vi "set gain and exp time for Basler acA2500-60um (SubVI).vi"(7 "Acquisition Control::Exposure Time":dbl, 8 "error in (no error)":errorcluster, 9 "Analog Control::Gain":dbl, 10 "Session Out":T2, 11 "Refnum in":T1) -> (0 "error out":errorcluster, 3 "Refnum out":T1)   [LabVIEW 2024]
uses:
  <vilib>/userDefined/High Color/IMAQdx.ctl
  <vilib>/vision/Image Controls.llb/IMAQ Image.ctl
  <resource>/objmgr/imaqdx.rc
  <vilib>/vision/driver/NI_Vision_Acquisition_Software.lvlib
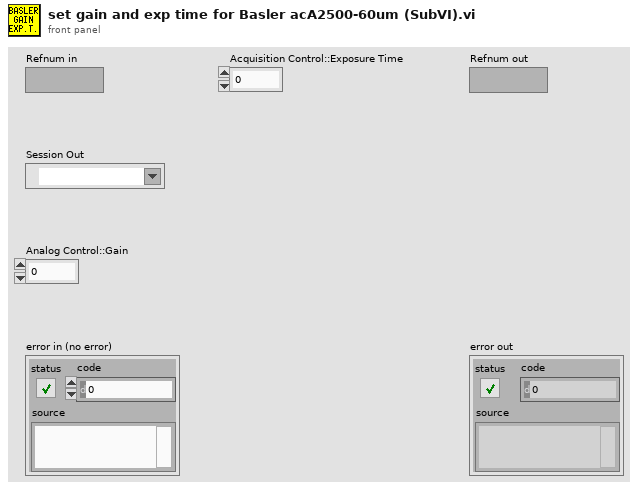
[diagram p1: front panel]
types:
  T1 = typedef "IMAQ Image.ctl" = refnum<image>
  T2 = typedef "IMAQdx.ctl" = refnum<k21>
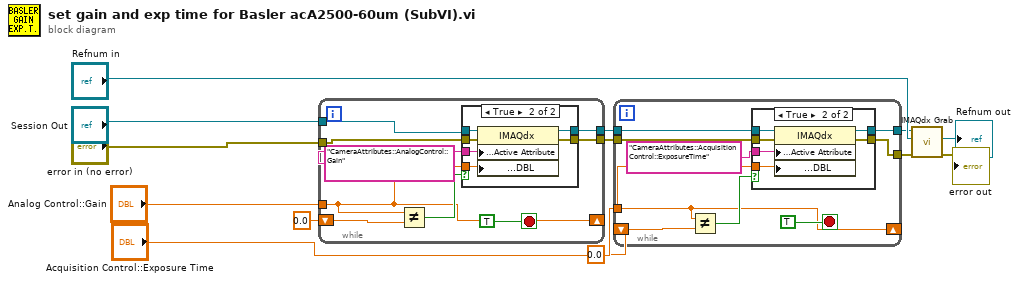
[diagram p0: block diagram]
diagram:
  n1 = while {
    tunnel: [w22] -> w4
    tunnel: [w21] -> w3
    shift-right: [w14] -> _
    shift-left: 0.0 ("Analog Control::Gain") -> [w18]
    tunnel: "Session Out" -> [w16]
    tunnel: "error in (no error)" -> [w15]
    tunnel: "Analog Control::Gain" -> [w14]
    stop <- TRUE stop-if-true
    n2 = Not Equal?(x=w14, y=w18) -> (x != y?=w17:bool)
    n3 = case shown="True" w17 {
      tunnel: w15 -> [w23 w30]
      tunnel: [w24 w29] -> w22
      tunnel: w16 -> [w24 w28]
      tunnel: [w23 w27] -> w21
      tunnel: "CameraAttributes::AnalogControl::Gain" ("Name") -> [_ w26]
      tunnel: w14 -> [_ w25]
      frame False {
      }
      frame True {
        n4 = property class="IMAQdx"(reference=w28, error in=w30, "Camera Attributes:Active Attribute"=w26, "Camera Attributes:Value:DBL"=w25) -> (reference out=w29:T2, error out=w27:errorcluster)
      }
    }
  }
  n5 = while {
    tunnel: w3 -> [w39]
    tunnel: [w38] -> w7
    tunnel: w4 -> [w37]
    tunnel: [w36] -> w5
    shift-right: [w31] -> _
    shift-left: 0.0 ("Acquisition Control::Exposure Time") -> [w33]
    tunnel: "Acquisition Control::Exposure Time" -> [w31]
    stop <- TRUE stop-if-true
    n6 = Not Equal?(x=w31, y=w33) -> (x != y?=w32:bool)
    n7 = case shown="True" w32 {
      tunnel: w39 -> [w40 w47]
      tunnel: [w41 w46] -> w38
      tunnel: w37 -> [w41 w45]
      tunnel: [w40 w44] -> w36
      tunnel: "CameraAttributes::AcquisitionControl::ExposureTime" ("Name") -> [_ w43]
      tunnel: w31 -> [_ w42]
      frame False {
      }
      frame True {
        n8 = property class="IMAQdx"(reference=w45, error in=w47, "Camera Attributes:Active Attribute"=w43, "Camera Attributes:Value:DBL"=w42) -> (reference out=w46:T2, error out=w44:errorcluster)
      }
    }
  }
  n9 = call <vilib>:"IMAQdx Grab.vi"("error in"=w5, "Image In"="Refnum in", "Session In"=w7) -> ("error out"=→"error out":errorcluster, "Image Out"=→"Refnum out":T1)  [unwired: 1 in, 6 out]
